vi "insert_image.vi"(8 "error in (no error)":errorcluster, 10 "image":refnum<class "Image.lvclass">, 11 "DataCollectionMG091001IntrinsicImaging in":refnum<class "DataCollectionMG091001IntrinsicImaging.lvclass">) -> (0 "error out":errorcluster, 3 "DataCollectionMG091001IntrinsicImaging out":refnum<class "DataCollectionMG091001IntrinsicImaging.lvclass">)   [LabVIEW 2010, in "DataCollectionMG091001IntrinsicImaging.lvclass"]
uses:
  DataCollectionMG091001IntrinsicImaging.lvclass
  common/classes/Image/Image/Image.lvclass
  DataCollectionMG091001IntrinsicImaging.lvclass/DataCollectionMG091001IntrinsicImaging.ctl
  common/classes/ImageCollection/ImageCollection/add_mode_enum.ctl
  common/classes/ImageCollection/ImageCollection/ImageCollection.lvclass
  common/classes/ErrorController/ErrorController/class_data.vi
  common/classes/ErrorController/ErrorController/ErrorController.lvclass
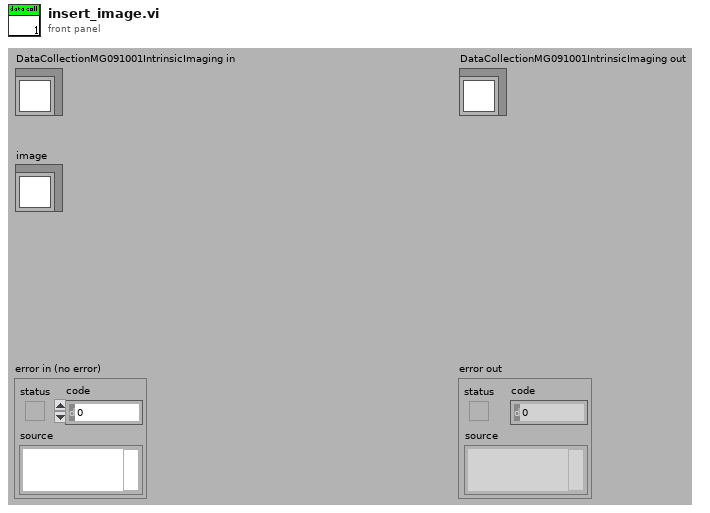
[diagram p1: front panel]
types:
  T1 = typedef "ImageCollection.lvclass/add_mode_enum.ctl" = enum16{"instance", "copy"}
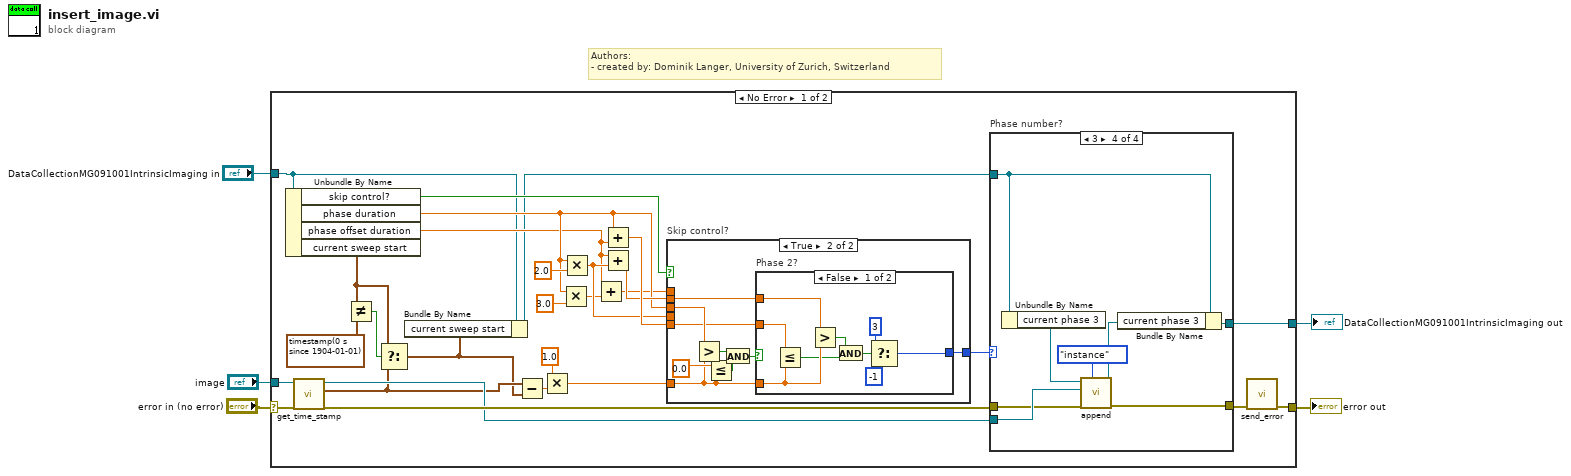
[diagram p0: block diagram]
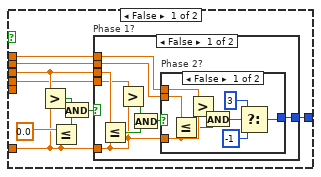
[diagram p2: hidden frame]
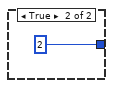
[diagram p3: hidden frame]
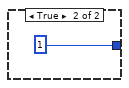
[diagram p4: hidden frame]
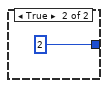
[diagram p5: hidden frame]
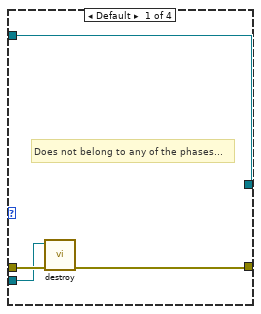
[diagram p6: hidden frame]
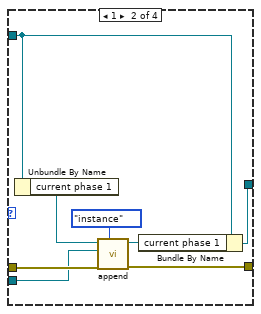
[diagram p7: hidden frame]
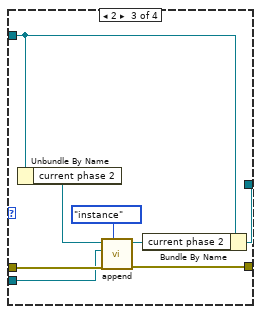
[diagram p8: hidden frame]
diagram:
  # "Authors: \n- created by: Dominik Langer, University of Zurich, Switzerland"
  n1 = case shown="No Error" "error in (no error)" {
    selector: "error in (no error)" -> [w33 w112]
    tunnel: [w7 w112] -> w4
    tunnel: [w23 w111] -> w2
    tunnel: "DataCollectionMG091001IntrinsicImaging in" -> [w12 w111]
    tunnel: "image" -> [w32 _]
    frame No Error {
      n2 = Unbundle By Name(w12) -> ("skip control?"=w30:bool, "phase duration"=w18:dbl[unit], "phase offset duration"=w17:dbl[unit], "current sweep start"=w8:timestamp)
      n3 = call-dynamic "get_time_stamp.vi"("error in (no error)"=w33, "Image.lvclass in"=w32) -> ("error out"=w24:errorcluster, "timestamp"=w14:timestamp, "Image.lvclass out"=w22:refnum<class "Image.lvclass">)  [unwired: 7 in]
      n4 = Not Equal?(x=w8, y=timestamp(0 s since 1904-01-01)) -> (x != y?=w13:bool)
      n5 = Select(t=w8, s=w13, f=w14) -> (s? t:f=w10:timestamp)
      n6 = Bundle By Name(cluster=w12, "current sweep start"=w10) -> (w11:refnum<class "DataCollectionMG091001IntrinsicImaging.lvclass">)
      n7 = Subtract(x=w14, y=w10) -> (x-y=w26:dbl)
      n8 = Multiply(x=dbl[unit] 1.0 ("y"), y=w26) -> (x*y=w29:dbl[unit])
      n9 = Multiply(x=w18, y=3.0) -> (x*y=w16:dbl[unit])
      n10 = Multiply(x=w18, y=2.0) -> (x*y=w20:dbl[unit])
      n11 = Add(x=w17, y=w16) -> (x+y=w15:dbl[unit])
      n12 = Add(x=w18, y=w17) -> (x+y=w28:dbl[unit])
      n13 = Add(x=w17, y=w20) -> (x+y=w25:dbl[unit])
      n14 = case "Skip control?" shown="True" w30 {
        tunnel: w29 -> [w34 w64]
        tunnel: w18 -> [w39 w67]
        tunnel: w28 -> [_ w66]
        tunnel: [w40 w68] -> w21
        tunnel: w25 -> [w37 w65]
        tunnel: w20 -> [w38 _]
        tunnel: w15 -> [w36 _]
        frame False {
          n15 = Greater?(x=w39, y=w34) -> (0:w43:bool)
          n16 = Less Or Equal?(x=dbl[unit] 0.0, y=w34) -> (x <= y?=w42:bool)
          n17 = And(x=w43, y=w42) -> (x .and. y?=w41:bool)
          n18 = case "Phase 1?" shown="False" w41 {
            tunnel: [w47 1] -> w40
            tunnel: w34 -> [w46 _]
            tunnel: w39 -> [w52 _]
            tunnel: w38 -> [w51 _]
            tunnel: w37 -> [w45 _]
            tunnel: w36 -> [w44 _]
            frame False {
              n19 = Less Or Equal?(x=w52, y=w46) -> (x <= y?=w50:bool)
              n20 = Greater?(x=w51, y=w46) -> (0:w49:bool)
              n21 = And(x=w49, y=w50) -> (x .and. y?=w48:bool)
              n22 = case "Phase 2?" shown="False" w48 {
                tunnel: [w53 2] -> w47
                tunnel: w46 -> [w59 _]
                tunnel: w45 -> [w61 _]
                tunnel: w44 -> [w60 _]
                frame False {
                  n23 = Less Or Equal?(x=w61, y=w59) -> (x <= y?=w58:bool)
                  n24 = Greater?(x=w60, y=w59) -> (0:w57:bool)
                  n25 = And(x=w57, y=w58) -> (x .and. y?=w56:bool)
                  n26 = Select(t=3, s=w56, f=-1) -> (s? t:f=w53:i32)
                }
                frame True {
                }
              }
            }
            frame True {
            }
          }
        }
        frame True {
          n27 = Greater?(x=w67, y=w64) -> (0:w71:bool)
          n28 = Less Or Equal?(x=dbl[unit] 0.0, y=w64) -> (x <= y?=w70:bool)
          n29 = And(x=w71, y=w70) -> (x .and. y?=w69:bool)
          n30 = case "Phase 2?" shown="False" w69 {
            tunnel: [w73 2 ("f")] -> w68
            tunnel: w64 -> [w79 _]
            tunnel: w66 -> [w81 _]
            tunnel: w65 -> [w80 _]
            frame False {
              n31 = Less Or Equal?(x=w81, y=w79) -> (x <= y?=w78:bool)
              n32 = Greater?(x=w80, y=w79) -> (0:w77:bool)
              n33 = And(x=w77, y=w78) -> (x .and. y?=w75:bool)
              n34 = Select(t=3, s=w75, f=-1) -> (s? t:f=w73:i32)
            }
            frame True {
            }
          }
        }
      }
      n35 = case "Phase number?" shown="3" w21 {
        tunnel: [w83 w92 w100 w108] -> w23
        tunnel: [w84 w94 w102 w110] -> w6
        tunnel: w24 -> [w86 w90 w96 w104]
        tunnel: w11 -> [w83 w88 w98 w103]
        tunnel: w22 -> [w85 w87 w95 w105]
        frame Default {
          # "Does not belong to any of the phases..."
          n36 = call-dynamic "destroy.vi"("error in (no error)"=w86, "Image in"=w85) -> ("error out"=w84:errorcluster)  [unwired: 8 in, 1 out]
        }
        frame 1 {
          n37 = Unbundle By Name(w88) -> ("current phase 1"=w89:refnum<class "ImageCollection.lvclass">)
          n38 = call-dynamic "append.vi"("add mode"=add_mode_enum."instance", "error in (no error)"=w90, "Image.lvclass"=w87, "ImageCollection in"=w89) -> ("error out"=w94:errorcluster, "ImageCollection out"=w91:refnum<class "ImageCollection.lvclass">)  [unwired: 5 in, 1 out]
          n39 = Bundle By Name(cluster=w88, "current phase 1"=w91) -> (w92:refnum<class "DataCollectionMG091001IntrinsicImaging.lvclass">)
        }
        frame 2 {
          n40 = Unbundle By Name(w98) -> ("current phase 2"=w97:refnum<class "ImageCollection.lvclass">)
          n41 = call-dynamic "append.vi"("add mode"=add_mode_enum."instance", "error in (no error)"=w96, "Image.lvclass"=w95, "ImageCollection in"=w97) -> ("error out"=w102:errorcluster, "ImageCollection out"=w99:refnum<class "ImageCollection.lvclass">)  [unwired: 5 in, 1 out]
          n42 = Bundle By Name(cluster=w98, "current phase 2"=w99) -> (w100:refnum<class "DataCollectionMG091001IntrinsicImaging.lvclass">)
        }
        frame 3 {
          n43 = Unbundle By Name(w103) -> ("current phase 3"=w106:refnum<class "ImageCollection.lvclass">)
          n44 = call-dynamic "append.vi"("add mode"=add_mode_enum."instance", "error in (no error)"=w104, "Image.lvclass"=w105, "ImageCollection in"=w106) -> ("error out"=w110:errorcluster, "ImageCollection out"=w107:refnum<class "ImageCollection.lvclass">)  [unwired: 5 in, 1 out]
          n45 = Bundle By Name(cluster=w103, "current phase 3"=w107) -> (w108:refnum<class "DataCollectionMG091001IntrinsicImaging.lvclass">)
        }
      }
      n46 = call "send_error.vi"("error in (no error)"=w6) -> ("error out"=w7:errorcluster)  [unwired: 10 in]
    }
    frame Error {
    }
  }
  "error out" <- w4
  "DataCollectionMG091001IntrinsicImaging out" <- w2
